vi "LittleBoatHindbrainSense.vi"(9 "output cluster":T3, 10 "XBee Serial Port":refnum<visa-resource-name>, 11 "connection ID":refnum<k16>) -> (0 "error out":errorcluster)   [LabVIEW 2013]
uses:
  Data/TypeDefs/GPS-Compass Queue Cluster.ctl
  Data/TypeDefs/UTM Location.ctl
  Data/TypeDefs/WindData Queue Cluster.ctl
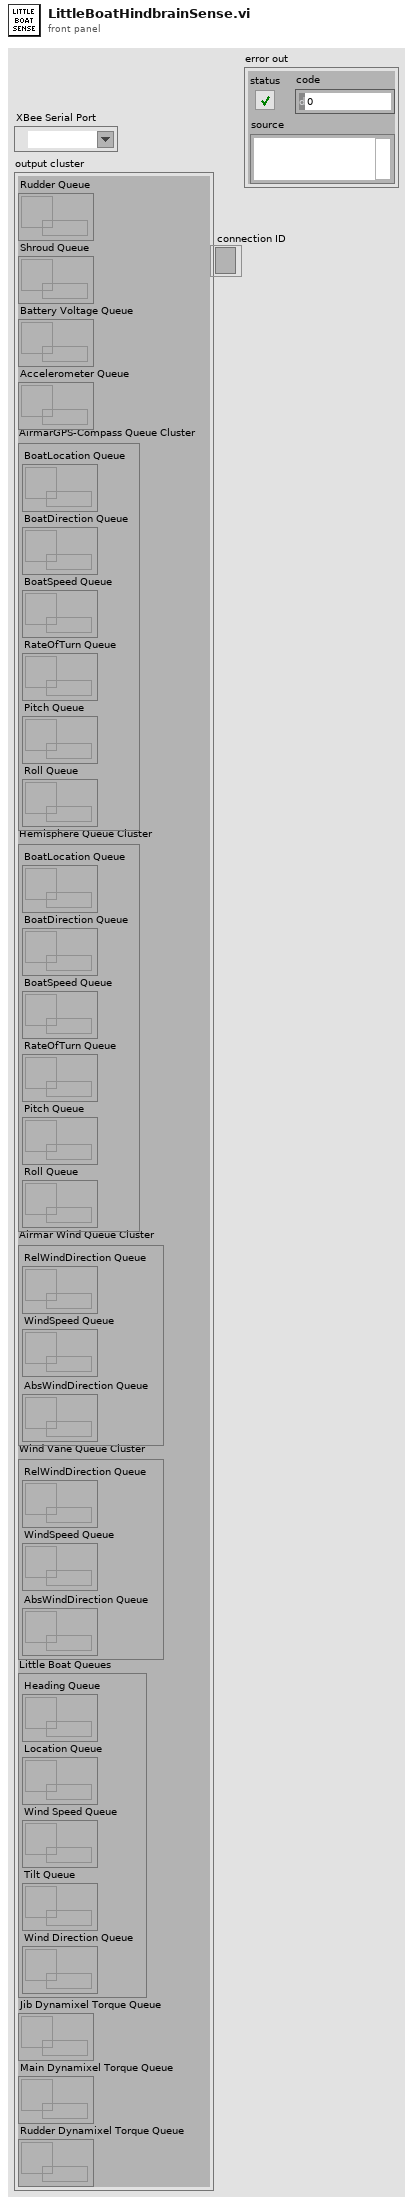
[diagram p1: front panel]
types:
  T1 = typedef "GPS-Compass Queue Cluster.ctl" = cluster{"BoatLocation Queue":refnum<queue>, "BoatDirection Queue":refnum<queue>, "BoatSpeed Queue":refnum<queue>, "RateOfTurn Queue":refnum<queue>, "Pitch Queue":refnum<queue>, "Roll Queue":refnum<queue>}
  T2 = typedef "WindData Queue Cluster.ctl" = cluster{"RelWindDirection Queue":refnum<queue>, "WindSpeed Queue":refnum<queue>, "AbsWindDirection Queue":refnum<queue>}
  T3 = cluster{"Rudder Queue":refnum<queue>, "Shroud Queue":refnum<queue>, "Battery Voltage Queue":refnum<queue>, "Accelerometer Queue":refnum<queue>, "AirmarGPS-Compass Queue Cluster":T1, "Hemisphere Queue Cluster":T1, "Airmar Wind Queue Cluster":T2, "Wind Vane Queue Cluster":T2, "Little Boat Queues":cluster{"Heading Queue":refnum<queue>, "Location Queue":refnum<queue>, "Wind Speed Queue":refnum<queue>, "Tilt Queue":refnum<queue>, "Wind Direction Queue":refnum<queue>}, "Jib Dynamixel Torque Queue":refnum<queue>, "Main Dynamixel Torque Queue":refnum<queue>, "Rudder Dynamixel Torque Queue":refnum<queue>}
  T4 = typedef "UTM Location.ctl" = cluster{"UTM Zone":dbl, "Hemisphere":enum16{"North", "South"}, "East":dbl, "North":dbl}
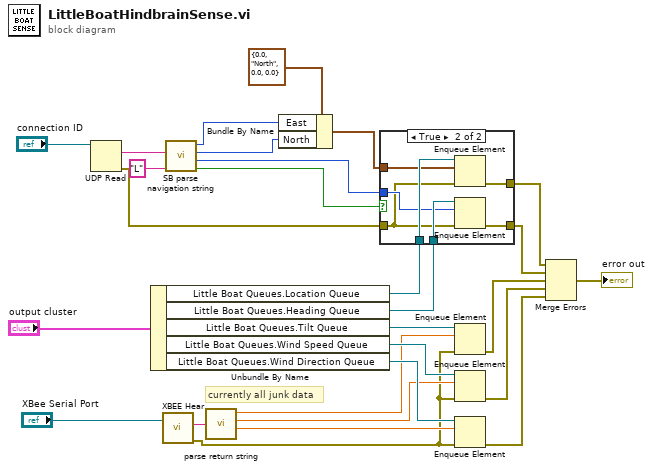
[diagram p0: block diagram]
diagram:
  # "currently all junk data"
  n1 = UDP Read(connection ID="connection ID") -> (data out=w8:string, error out=w1:errorcluster)  [unwired: 3 in, 3 out]
  n2 = Unbundle By Name("output cluster") -> ("Little Boat Queues.Location Queue"=w16:refnum<queue>, "Little Boat Queues.Heading Queue"=w15:refnum<queue>, "Little Boat Queues.Tilt Queue"=w17:refnum<queue>, "Little Boat Queues.Wind Speed Queue"=w19:refnum<queue>, "Little Boat Queues.Wind Direction Queue"=w21:refnum<queue>)
  n3 = call "XBEE Hear.vi"("VISA resource name"="XBee Serial Port") -> ("String Received"=w13:string, "error out"=w11:errorcluster)  [unwired: 1 in, 2 out]
  n4 = call "SB parse navigation string.vi"("Header"="L" ("Tug"), "Nav String"=w8) -> ("Valid?"=w7:bool, "angle"=w6:i32, "y"=w3:i32, "x"=w4:i32)  [unwired: 4 in]
  n5 = call "parse return string.vi"("Return String"=w13) -> ("Tilt"=w18:dbl, "Wind Speed"=w20:dbl, "Wind Direction"=w22:dbl)  [unwired: 1 out]
  n6 = Bundle By Name(cluster=T4 {"UTM Zone"=0.0, "Hemisphere"=enum."North", "East"=0.0, "North"=0.0} ("UTM Location"), "East"=w4, "North"=w3) -> (w2:T4)
  n7 = case shown="True" w7 {
    tunnel: [w29 w36] -> w25
    tunnel: [w29 w35] -> w24
    tunnel: w16 -> [_ w34]
    tunnel: w15 -> [_ w33]
    tunnel: w6 -> [_ w32]
    tunnel: w2 -> [_ w31]
    tunnel: w1 -> [w29 w30]
    frame False {
    }
    frame True {
      n8 = Enqueue Element(queue=w34, element=w31, error in (no error)=w30) -> (error out=w35:errorcluster)  [unwired: 1 in, 2 out]
      n9 = Enqueue Element(queue=w33, element=w32, error in (no error)=w30) -> (error out=w36:errorcluster)  [unwired: 1 in, 2 out]
    }
  }
  n10 = Enqueue Element(queue=w17, element=w18, error in (no error)=w11) -> (error out=w26:errorcluster)  [unwired: 1 in, 2 out]
  n11 = Enqueue Element(queue=w19, element=w20, error in (no error)=w11) -> (error out=w27:errorcluster)  [unwired: 1 in, 2 out]
  n12 = Enqueue Element(queue=w21, element=w22, error in (no error)=w11) -> (error out=w28:errorcluster)  [unwired: 1 in, 2 out]
  n13 = Merge Errors(w24, w25, w26, w27, w28) -> (→"error out":errorcluster)
